vi "DAQ.EnumerateAndSortDevices.vi"(8 "error in (no error)":errorcluster, 11 "Instrument.DAQ":refnum<class "Instrument.DAQ.lvclass">) -> (0 "error out":errorcluster, 2 "Devices (sorted)":T1[](array[typedef])=[{"DeviceName"="PXI1Slot5", "DevIsSimulated"=FALSE, "DeviceSerialNumber"=21267641, "ProductType"="PXI-4461", "ProductCategory"=14649, "ProductNumber"=29299, "ChassisNumber"=1, "SlotNumber"=5, "ChassisName"="NI PXIe-1082DC", "ChassisSerialNumber"=50979316}, {"DeviceName"="PXI1Slot6", "DevIsSimulated"=FALSE, "DeviceSerialNumber"=21267639, "ProductType"="PXI-4461", "ProductCategory"=14649, "ProductNumber"=29299, "ChassisNumber"=1, "SlotNumber"=6, "ChassisName"="NI PXIe-1082DC", "ChassisSerialNumber"=50979316}, {"DeviceName"="PXI1Slot7", "DevIsSimulated"=FALSE, "DeviceSerialNumber"=20037036, "ProductType"="PXI-4461", "ProductCategory"=14649, "ProductNumber"=29299, "ChassisNumber"=1, "SlotNumber"=7, "ChassisName"="NI PXIe-1082DC", "ChassisSerialNumber"=50979316}, {"DeviceName"="PXI1Slot8", "DevIsSimulated"=FALSE, "DeviceSerialNumber"=20037044, "ProductType"="PXI-4461", "ProductCategory"=14649, "ProductNumber"=29299, "ChassisNumber"=1, "SlotNumber"=8, "ChassisName"="NI PXIe-1082DC", "ChassisSerialNumber"=50979316}, {"DeviceName"="Dev1", "DevIsSimulated"=FALSE, "DeviceSerialNumber"=0, "ProductType"="", "ProductCategory"=0, "ProductNumber"=0, "ChassisNumber"=4294967295, "SlotNumber"=0, "ChassisName"="", "ChassisSerialNumber"=0}], 3 "Instrument.DAQ out":refnum<class "Instrument.DAQ.lvclass">)   [LabVIEW 2019, in "Instrument.Lockin.lvlib" / "Instrument.DAQ.lvclass"]
uses:
  Instrument.DAQ.lvclass
  Typedefs/DeviceInfo--Cluster.ctl
  Instrument.DAQ.lvclass/Instrument.DAQ.ctl
  <userlib>/_OpenG.lib/array/array.llb/Sort 1D Array (U32)__ogtk.vi
  <userlib>/_OpenG.lib/array/array.llb/Reorder 1D Array2 (Variant)__ogtk.vi
  <vilib>/numeric/Random Number (Range) I64.vi
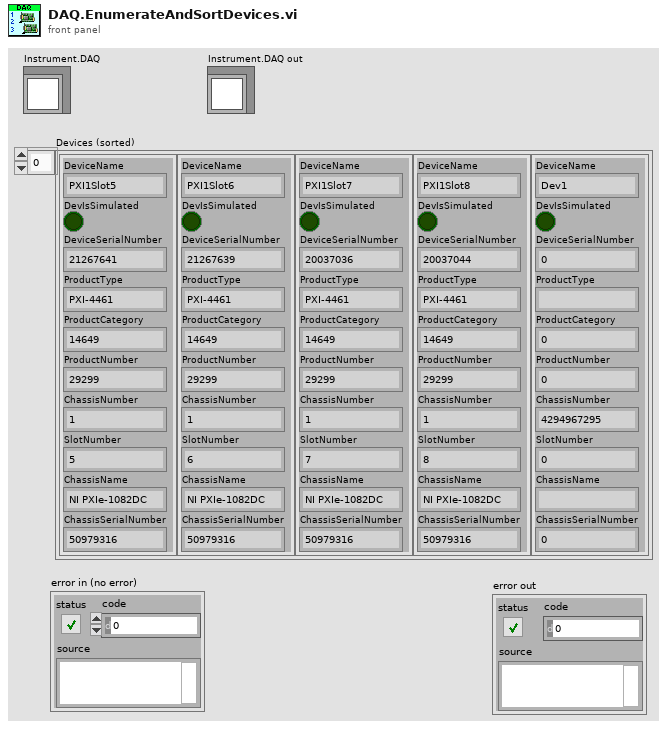
[diagram p1: front panel]
types:
  T1 = typedef "Instrument.Lockin.lvlib/Instrument.DAQ.lvclass/DeviceInfo--Cluster.ctl" = cluster{"DeviceName":string, "DevIsSimulated":bool, "DeviceSerialNumber":u32, "ProductType":string, "ProductCategory":i32, "ProductNumber":u32, "ChassisNumber":u32, "SlotNumber":u32, "ChassisName":string, "ChassisSerialNumber":u32}
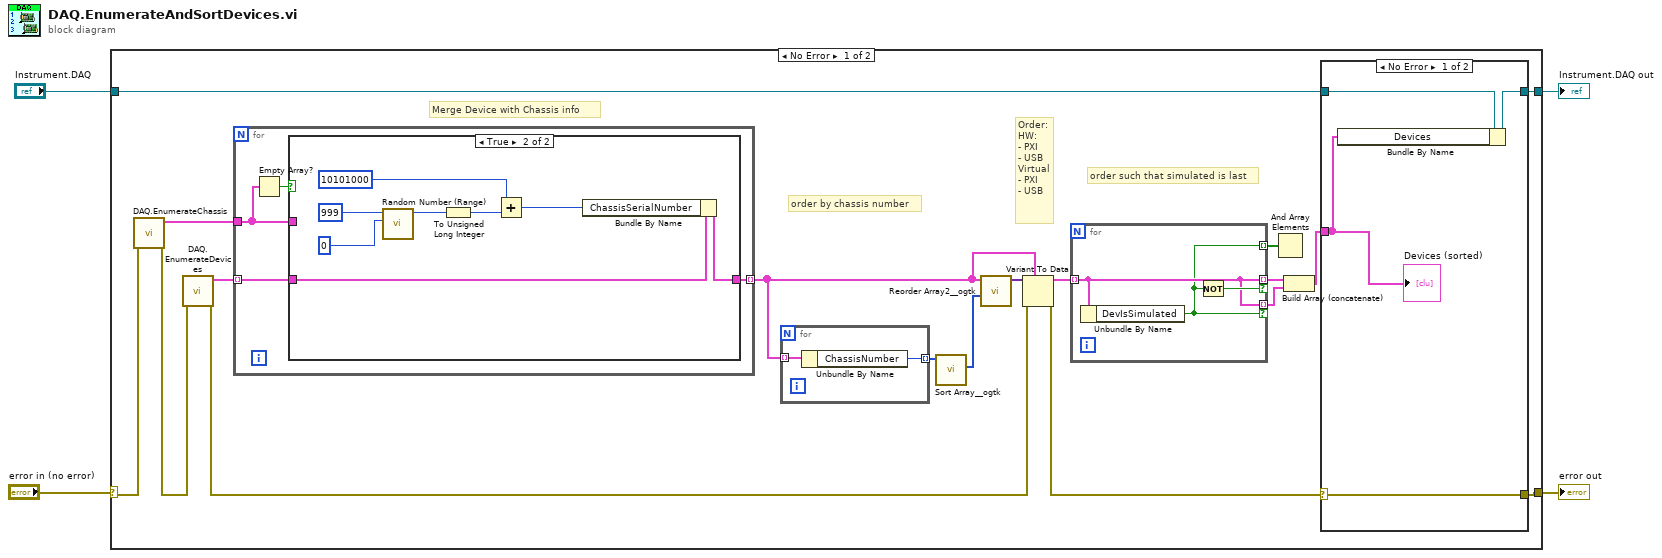
[diagram p0: block diagram]
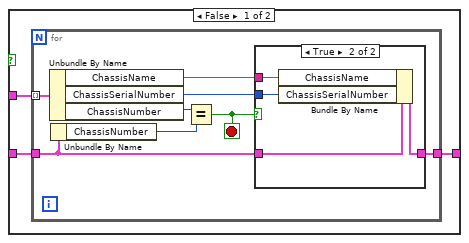
[diagram p2: hidden frame]
diagram:
  n1 = case shown="No Error" "error in (no error)" {
    selector: "error in (no error)" -> [w7 w63]
    tunnel: [w13 w63] -> w3
    tunnel: "Instrument.DAQ" -> [w10 w62]
    tunnel: [w11 w62] -> w1
    frame No Error {
      # "Order:\nHW:\n- PXI\n- USB\nVirtual\n- PXI\n- USB"
      # "order by chassis number"
      # "order such that simulated is last"
      # "Merge Device with Chassis info"
      n2 = call "DAQ.EnumerateChassis.vi"("error in (no error)"=w7) -> ("error out"=w6:errorcluster, "Chassis"=w19:T1[])  [unwired: 9 in]
      n3 = call "DAQ.EnumerateDevices.vi"("error in (no error)"=w6) -> ("error out"=w5:errorcluster, "Devices"=w20:T1[])  [unwired: 9 in]
      n4 = for {
        tunnel: w19 -> [w24]
        tunnel: w20 -> [w25] mode=indexing
        tunnel: [w26] -> w15 mode=indexing
        n5 = Empty Array?(array=w24) -> (empty?=w23:bool)
        n6 = case shown="True" w23 {
          tunnel: [w29 w50] -> w26
          tunnel: w25 -> [w28 w49]
          tunnel: w24 -> [w27 _]
          frame False {
            n7 = for {
              tunnel: w28 -> [w30]
              tunnel: w27 -> [w37] mode=indexing
              tunnel: [w32] -> w29
              stop <- w31 stop-if-true
              n8 = Unbundle By Name(w37) -> ("ChassisName"=w34:string, "ChassisSerialNumber"=w33:u32, "ChassisNumber"=w36:u32)
              n9 = Unbundle By Name(w30) -> ("ChassisNumber"=w35:u32)
              n10 = Equal?(x=w36, y=w35) -> (x = y?=w31:bool)
              n11 = case shown="True" w31 {
                tunnel: w30 -> [w38 w42]
                tunnel: w34 -> [_ w41]
                tunnel: w33 -> [_ w39]
                tunnel: [w38 w40] -> w32
                frame False {
                }
                frame True {
                  n12 = Bundle By Name(cluster=w42, "ChassisName"=w41, "ChassisSerialNumber"=w39) -> (w40:T1)
                }
              }
            }
          }
          frame True {
            n13 = call-poly <vilib>:"Random Number (Range).vi"("lower bound (-100)"=i64 0, "upper bound (100)"=i64 999) -> ("number"=w44:i64)  [unwired: 9 in]
            n14 = To Unsigned Long Integer(number=w44) -> (unsigned 32bit integer=w43:u32)
            n15 = Add(x=u32 10101000 ("ChassisSerialNumber"), y=w43) -> (x+y=w45:u32)
            n16 = Bundle By Name(cluster=w49, "ChassisSerialNumber"=w45) -> (w50:T1)
          }
        }
      }
      n17 = for {
        tunnel: w15 -> [w55] mode=indexing
        tunnel: [w54] -> w18 mode=indexing
        n18 = Unbundle By Name(w55) -> ("ChassisNumber"=w54:u32)
      }
      n19 = call-poly <userlib>:"Sort Array__ogtk.vi"("Array in"=w18) -> ("Sorted Pointers"=w17:i32[])  [unwired: 9 in, 1 out]
      n20 = call-poly <userlib>:"Reorder Array2__ogtk.vi"("indices"=w17, "array"=w15) -> ("reordered array"=w16:variant[])  [unwired: 9 in]
      n21 = Variant To Data(error in=w5, type=w15, Variant=w16) -> (data=w14:T1[], error out=w12:errorcluster)
      n22 = for {
        tunnel: [w52] -> w22 mode=indexing if=w53
        tunnel: w14 -> [w52] mode=indexing
        tunnel: [w52] -> w21 mode=indexing if=w51
        tunnel: [w51] -> w9 mode=indexing
        n23 = Unbundle By Name(w52) -> ("DevIsSimulated"=w51:bool)
        n24 = Not(x=w51) -> (.not. x?=w53:bool)
      }
      n25 = And Array Elements(Boolean array=w9) -> ()  [unwired: 1 out]
      n26 = Build Array (concatenate)(w22, w21) -> (w8:T1[])
      n27 = case shown="No Error" w12 {
        selector: w12 -> [w59 w60]
        tunnel: [w59 w60] -> w13
        tunnel: [w57 w61] -> w11
        tunnel: w10 -> [w58 w61]
        tunnel: w8 -> [w56 _]
        frame No Error {
          n28 = Bundle By Name(cluster=w58, "Devices"=w56) -> (w57:refnum<class "Instrument.DAQ.lvclass">)
          "Devices (sorted)" <- w56
        }
        frame Error {
        }
      }
    }
    frame Error {
    }
  }
  "error out" <- w3
  "Instrument.DAQ out" <- w1
